vi "Info.vi"(8 "Error In":errorcluster, 11 "Text":string) -> (0 "Error Out":errorcluster)   [LabVIEW 2014, in "LV-Logger.lvlib"]
uses:
  LV-Logger.lvlib
  Private/Action.ctl
  Private/Message.ctl
  Private/Level.ctl
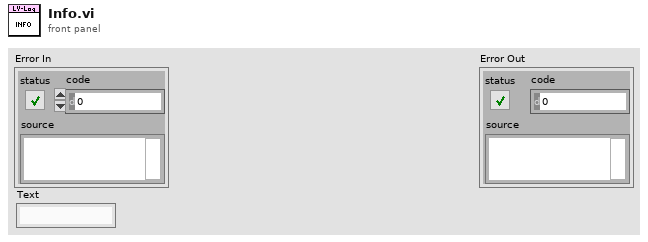
[diagram p1: front panel]
types:
  T1 = typedef "LV-Logger.lvlib/Level.ctl" = enum16{"Fatal", "Error", "Warn", "Info", "Debug", "Trace"}
  T2 = typedef "LV-Logger.lvlib/Action.ctl" = enum16{"Initialize", "Register", "Log", "Unregister", "Shutdown"}
  T3 = typedef "LV-Logger.lvlib/Message.ctl" = cluster{"Time Stamp":timestamp, "Level":T1, "Source":string, "Text":string}
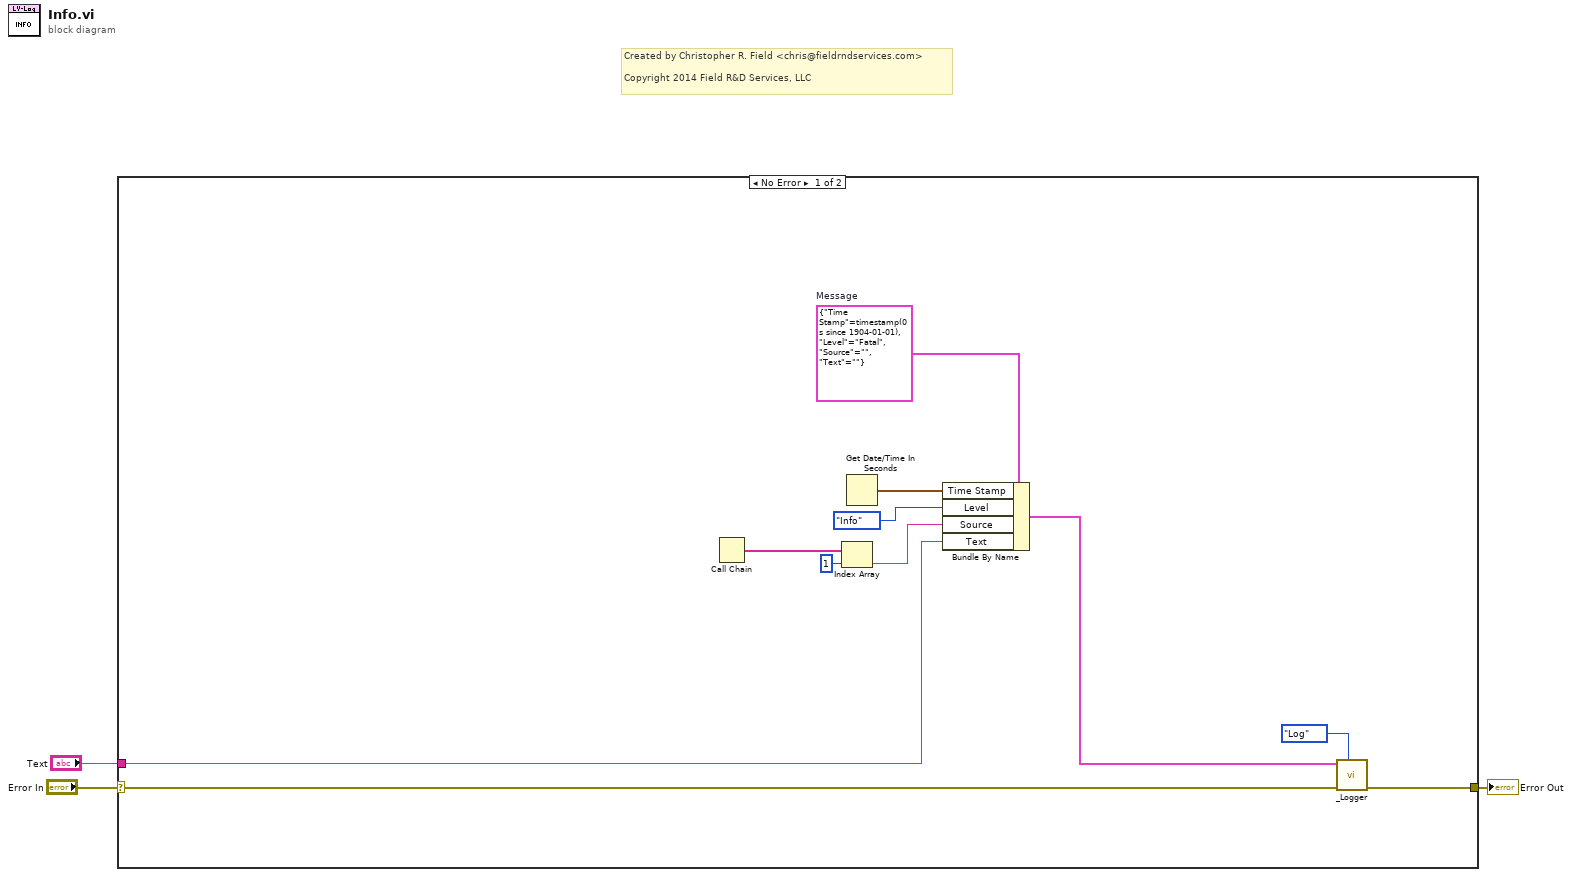
[diagram p0: block diagram]
diagram:
  # "Created by Christopher R. Field <chris@fieldrndservices.com>\n\nCopyright 2014 Field R&D Services, LLC"
  n1 = case shown="No Error" "Error In" {
    selector: "Error In" -> [w6 w15]
    tunnel: "Text" -> [w4 _]
    tunnel: [w5 w15] -> w1
    frame No Error {
      w11 = T3 {"Time Stamp"=timestamp(0 s since 1904-01-01), "Level"=enum."Fatal", "Source"="", "Text"=""}  # Message
      n2 = Call Chain() -> (call chain=w13:string[])
      n3 = Index Array(array=w13, index=1) -> (element=w8:string)
      n4 = Get Date/Time In Seconds() -> (seconds since 1Jan1904=w10:timestamp)
      n5 = Bundle By Name(cluster=w11, "Time Stamp"=w10, "Level"=Level."Info", "Source"=w8, "Text"=w4) -> (w7:T3)
      n6 = call "_Logger.vi"("Action"=Action."Log", "Error In"=w6, "Value In"=w7) -> ("Error Out"=w5:errorcluster)  [unwired: 8 in]
    }
    frame Error {
    }
  }
  "Error Out" <- w1
